vi "defects text.vi"(1 "info array":dbl[][](array[numeric]), 5 "pallet number":i16, 7 "curv num":i32, 9 "Start Button":bool, 11 "error in":errorcluster) -> (4 "defects:":string, 6 "This VI":refnum<vi>, 15 "error out":errorcluster)   [LabVIEW 2019]
panel:
  in  "Remove Button":bool
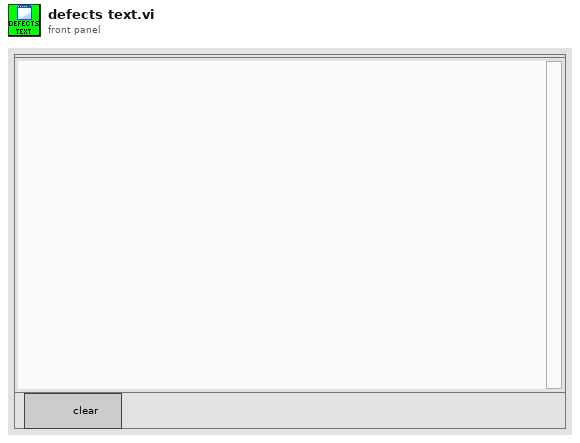
[diagram p1: front panel]
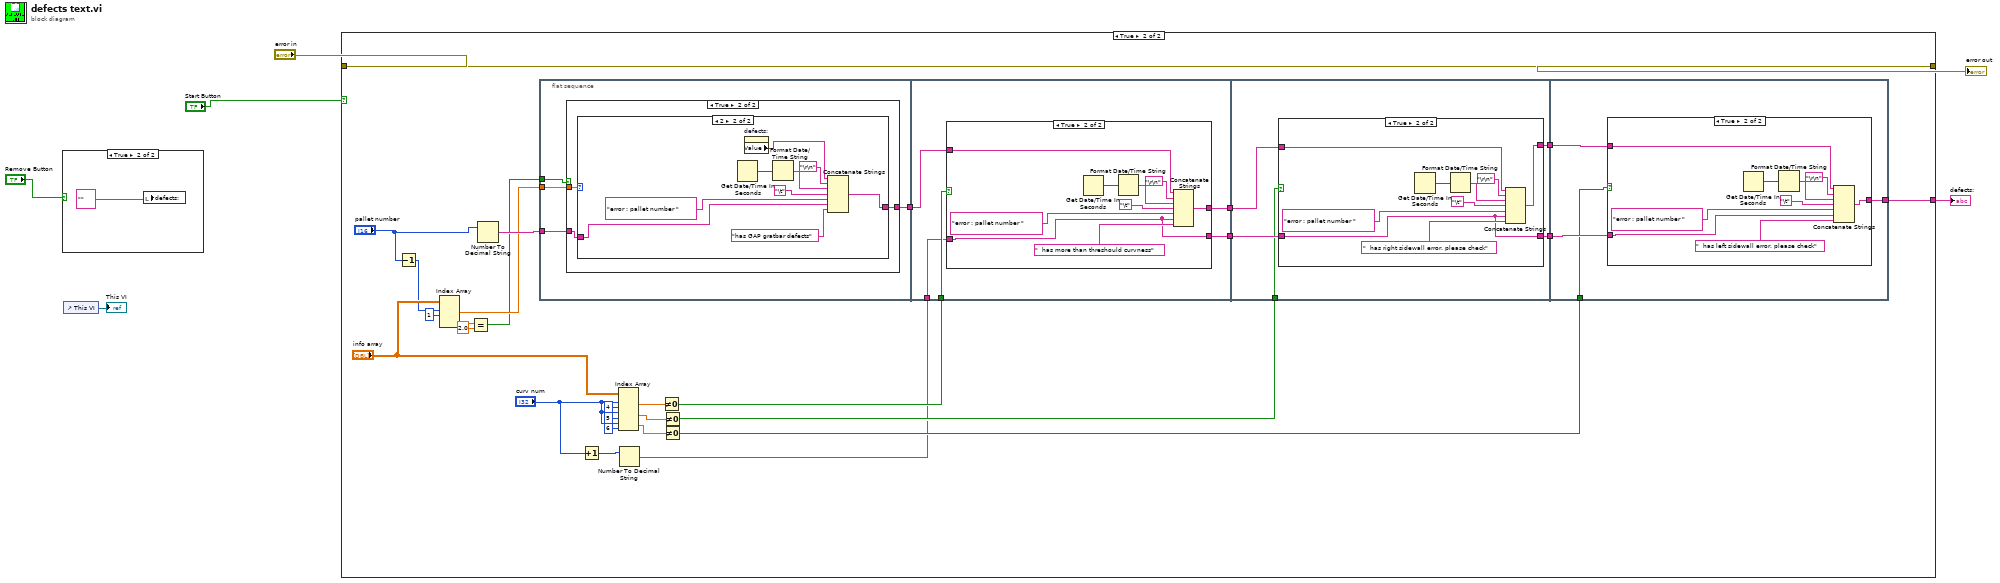
[diagram p0: block diagram]
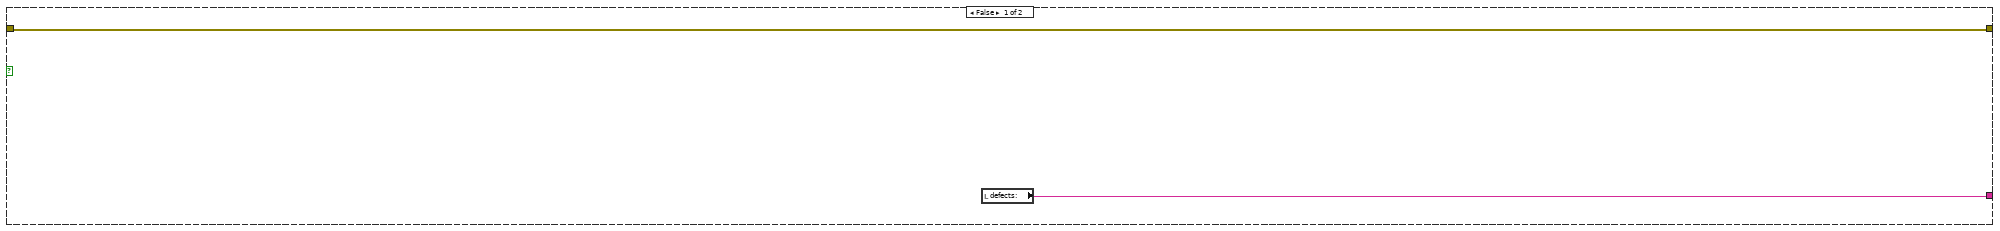
[diagram p3: hidden frame]
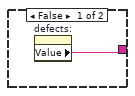
[diagram p4: hidden frame]
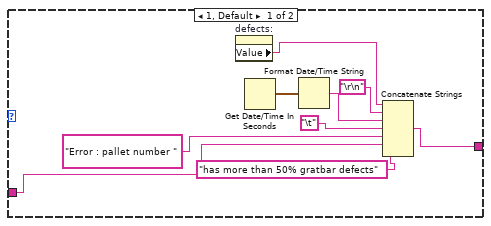
[diagram p5: hidden frame]
diagram:
  n1 = case shown="True" "Remove Button" {
    frame False {
    }
    frame True {
      n2 = local write "defects:"("" ("defects:")) -> ()
    }
  }
  n3 = control-ref of="This VI"() -> (→"This VI":refnum<vi>)
  n4 = case shown="True" "Start Button" {
    tunnel: [w9 w30] -> w4
    tunnel: [w8 w36] -> w3
    tunnel: "error in" -> [w8 w36]
    frame False {
      n5 = local read "defects:"() -> (w9:string)
    }
    frame True {
      n6 = Decrement(x="pallet number") -> (x-1=w14:i16)
      n7 = Index Array(array="info array", index (row) #1=w14, index (col) #1=1 ("disabled index (col)")) -> (element #1=w13:dbl, element #2=w12:dbl)  [unwired: 2 in]
      n8 = Equal?(x=w12, y=2.0) -> (x = y?=w10:bool)
      n9 = Number To Decimal String(number="pallet number") -> (decimal integer string=w37:string)  [unwired: 1 in]
      n10 = flat-sequence {
        tunnel: w13 -> [w41]
        tunnel: w37 -> [w40]
        tunnel: [w39] -> w35
        tunnel: w10 -> [w38]
        tunnel: w35 -> [w68]
        tunnel: [w67] -> w34
        tunnel: [w66] -> w33
        tunnel: w25 -> [w65]
        tunnel: w18 -> [w64]
        tunnel: w34 -> [w84]
        tunnel: w33 -> [w83]
        tunnel: [w82] -> w32
        tunnel: [w81] -> w31
        tunnel: w22 -> [w80]
        tunnel: w32 -> [w99]
        tunnel: w31 -> [w98]
        tunnel: [w97] -> w30
        tunnel: w21 -> [w96]
        frame #0 {
          n11 = case shown="True" w38 {
            tunnel: w41 -> [_ w45]
            tunnel: w40 -> [_ w44]
            tunnel: [w42 w43] -> w39
            frame False {
              n12 = property on="defects:" class="Str"() -> ("Value"=w42:string)  [unwired: 2 in, 2 out]
            }
            frame True {
              n13 = case shown="2" w45 {
                tunnel: w44 -> [w48 w57]
                tunnel: [w47 w56] -> w43
                frame 1, Default {
                  n14 = property on="defects:" class="Str"() -> ("Value"=w46:string)  [unwired: 2 in, 2 out]
                  n15 = Get Date/Time In Seconds() -> (seconds since 1Jan1904=w53:timestamp)
                  n16 = Format Date/Time String(seconds (now)=w53) -> (date/time string=w54:string)  [unwired: 2 in]
                  n17 = Concatenate Strings(w46, "\r\n", w54, "\t", "Error : pallet number " ("string"), w48, "has more than 50% gratbar defects" ("string")) -> (w47:string)
                }
                frame 2 {
                  n18 = Get Date/Time In Seconds() -> (seconds since 1Jan1904=w62:timestamp)
                  n19 = property on="defects:" class="Str"() -> ("Value"=w55:string)  [unwired: 2 in, 2 out]
                  n20 = Format Date/Time String(seconds (now)=w62) -> (date/time string=w63:string)  [unwired: 2 in]
                  n21 = Concatenate Strings(w55, "\r\n", w63, "\t", "error : pallet number " ("string"), w57, "has GAP gratbar defects" ("string")) -> (w56:string)
                }
              }
            }
          }
        }
        frame #1 {
          n22 = case shown="True" w65 {
            tunnel: w68 -> [w70 w73]
            tunnel: w64 -> [w69 w71]
            tunnel: [w70 w72] -> w67
            tunnel: [w69 w71] -> w66
            frame False {
            }
            frame True {
              n23 = Get Date/Time In Seconds() -> (seconds since 1Jan1904=w77:timestamp)
              n24 = Format Date/Time String(seconds (now)=w77) -> (date/time string=w75:string)  [unwired: 2 in]
              n25 = Concatenate Strings(w73, "\r\n", w75, "\t", "error : pallet number " ("string"), w71, "  has more than threshould curvness" ("string")) -> (w72:string)
            }
          }
        }
        frame #2 {
          n26 = case shown="True" w80 {
            tunnel: w84 -> [w86 w89]
            tunnel: w83 -> [w85 w87]
            tunnel: [w86 w88] -> w82
            tunnel: [w85 w87] -> w81
            frame False {
            }
            frame True {
              n27 = Get Date/Time In Seconds() -> (seconds since 1Jan1904=w93:timestamp)
              n28 = Format Date/Time String(seconds (now)=w93) -> (date/time string=w91:string)  [unwired: 2 in]
              n29 = Concatenate Strings(w89, "\r\n", w91, "\t", "error : pallet number " ("string"), w87, "  has right sidewall error. please check" ("string")) -> (w88:string)
            }
          }
        }
        frame #3 {
          n30 = case shown="True" w96 {
            tunnel: w99 -> [w100 w103]
            tunnel: w98 -> [_ w102]
            tunnel: [w100 w101] -> w97
            frame False {
            }
            frame True {
              n31 = Get Date/Time In Seconds() -> (seconds since 1Jan1904=w107:timestamp)
              n32 = Format Date/Time String(seconds (now)=w107) -> (date/time string=w105:string)  [unwired: 2 in]
              n33 = Concatenate Strings(w103, "\r\n", w105, "\t", "error : pallet number " ("string"), w102, "  has left sidewall error. please check" ("string")) -> (w101:string)
            }
          }
        }
      }
      n34 = Increment(x="curv num") -> (x+1=w19:i32)
      n35 = Index Array(array="info array", index (row) #1="curv num", index (col) #1=4 ("disabled index (col)"), index (row) #2="curv num", index (col) #2=5 ("disabled index (col)"), index (row) #3="curv num", index (col) #3=6 ("disabled index (col)")) -> (element #1=w29:dbl, element #2=w24:dbl, element #3=w23:dbl)
      n36 = Number To Decimal String(number=w19) -> (decimal integer string=w18:string)  [unwired: 1 in]
      n37 = Not Equal To 0?(x=w29) -> (x != 0?=w25:bool)
      n38 = Not Equal To 0?(x=w24) -> (x != 0?=w22:bool)
      n39 = Not Equal To 0?(x=w23) -> (x != 0?=w21:bool)
    }
  }
  "error out" <- w3
  "defects:" <- w4
